vi "Configure.vi"(8 "error in (no error)":errorcluster, 11 "DemoLasers in":refnum<class "DemoLasers.lvclass">) -> (0 "error out":errorcluster, 3 "DemoLasers out":refnum<class "DemoLasers.lvclass">)   [LabVIEW 2020, in "DemoLasers.lvlib" / "DemoLasers.lvclass"]
uses:
  DemoLasers.lvclass
  Hardware Abstraction Layer/Component/Laser/Laser/Laser.lvclass
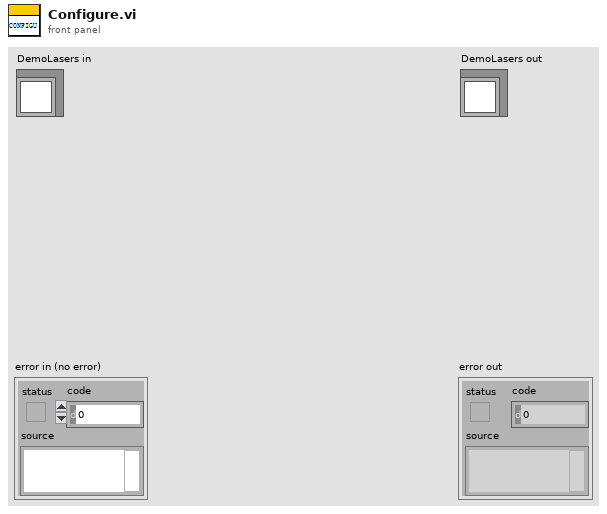
[diagram p1: front panel]
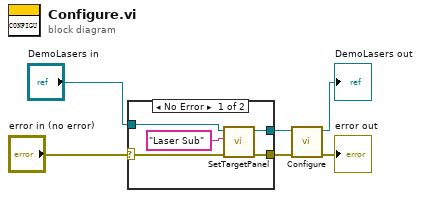
[diagram p0: block diagram]
diagram:
  n1 = case shown="No Error" "error in (no error)" {
    selector: "error in (no error)" -> [w10 w13]
    tunnel: [w9 w13] -> w1
    tunnel: [w7 w12] -> w2
    tunnel: "DemoLasers in" -> [w11 w12]
    frame No Error {
      n2 = call-dynamic "SetTargetPanel.vi"("error in (no error)"=w10, "TargetPanel"="Laser Sub" ("Sub Panel"), "GRMActor in"=w11) -> ("error out"=w9:errorcluster, "GRMActor out"=w7:refnum<class "DemoLasers.lvclass">)  [unwired: 7 in]
    }
    frame Error {
    }
  }
  n3 = call-parent "Configure.vi"("error in (no error)"=w1, "Device in"=w2) -> ("error out"=→"error out":errorcluster, "Device out"=→"DemoLasers out":refnum<class "DemoLasers.lvclass">)  [unwired: 8 in]
